vi "OverlayLibraryIconOnVI.vi"(8 "error in (no error)":errorcluster, 9 "Icon in":refnum<class "Icon.lvclass">, 10 "VI Refnum out":refnum<vi>, 11 "LVClassLibrary":refnum<vi>) -> (0 "error out":errorcluster, 1 "Icon out":refnum<class "Icon.lvclass">, 2 "VI Refnum out":refnum<vi>, 3 "LVClassLibrary":refnum<vi>)   [LabVIEW 2019, in "BlueUtilityScripts.lvlib"]
uses:
  <vilib>/LabVIEW Icon API/lv_icon/Classes/Icon/Icon.lvclass
  <vilib>/LabVIEW Icon API/API_User Layer Data.ctl
  <vilib>/Utility/miscctls.llb/LVPoint32TypeDef.ctl
  <vilib>/picture/picture.llb/imagedata.ctl
  BlueUtilityScripts.lvlib
  <vilib>/LabVIEW Icon API/LabVIEW Icon API.lvlib
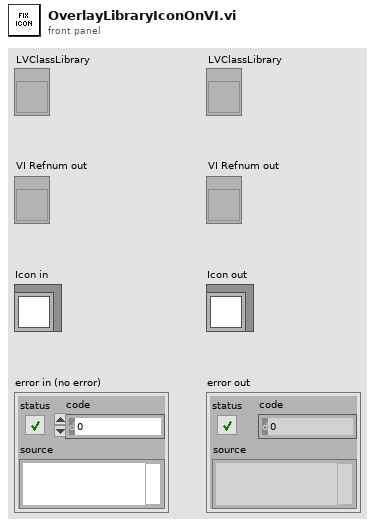
[diagram p1: front panel]
types:
  T1 = typedef "LVPoint32TypeDef.ctl" = cluster{"Horizontal":i32, "Vertical":i32}
  T2 = typedef "LabVIEW Icon API.lvlib/API_User Layer Data.ctl" = cluster{"Layer name":string, "Origin":T1, "Icon image data":T3}
  T3 = typedef "imagedata.ctl" = cluster{"image type":i32, "image depth":i32, "image":u8[], "mask":u8[], "colors":u32[], "Rectangle":cluster{"left":i16, "top":i16, "right":i16, "bottom":i16}}
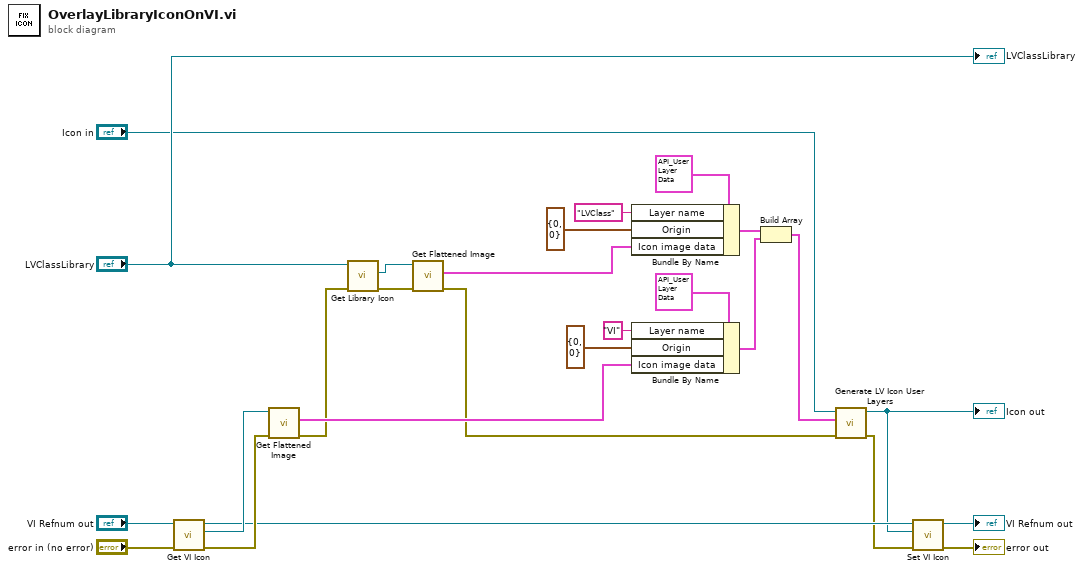
[diagram p0: block diagram]
diagram:
  n1 = call <vilib>:"Get VI Icon.vi"("error in (no error)"="error in (no error)", "VI Refnum in"="VI Refnum out") -> ("error out"=w12:errorcluster, "Icon"=w26:refnum<class "Icon.lvclass">, "VI Refnum out"=w5:refnum<vi>)  [unwired: 7 in]
  n2 = call <vilib>:"Get Flattened Image.vi"("error in (no error)"=w12, "lv_icon.lvlib:Icon.lvclass in"=w26) -> ("error out"=w10:errorcluster, "Color Image"=w15:T3)  [unwired: 6 in, 2 out]
  n3 = call <vilib>:"Get Library Icon.vi"("error in (no error)"=w10, "Library Refnum in"="LVClassLibrary") -> ("error out"=w11:errorcluster, "Icon"=w25:refnum<class "Icon.lvclass">)  [unwired: 7 in, 1 out]
  n4 = call <vilib>:"Get Flattened Image.vi"("error in (no error)"=w11, "lv_icon.lvlib:Icon.lvclass in"=w25) -> ("error out"=w9:errorcluster, "Color Image"=w19:T3)  [unwired: 6 in, 2 out]
  n5 = Bundle By Name(cluster=T2 {"Layer name"="", "Origin"={"Horizontal"=0, "Vertical"=0}, "Icon image data"={"image type"=0, "image depth"=0, "image"=[], "mask"=[], "colors"=[], "Rectangle"={"left"=0, "top"=0, "right"=0, "bottom"=0}}} ("User layer"), "Layer name"="LVClass", "Origin"=T1 {"Horizontal"=0, "Vertical"=0}, "Icon image data"=w19) -> (w21:T2)
  n6 = Bundle By Name(cluster=T2 {"Layer name"="", "Origin"={"Horizontal"=0, "Vertical"=0}, "Icon image data"={"image type"=0, "image depth"=0, "image"=[], "mask"=[], "colors"=[], "Rectangle"={"left"=0, "top"=0, "right"=0, "bottom"=0}}} ("User layer"), "Layer name"="VI", "Origin"=T1 {"Horizontal"=0, "Vertical"=0}, "Icon image data"=w15) -> (w14:T2)
  n7 = Build Array(w21, w14) -> (w20:T2[])
  n8 = call <vilib>:"Generate LV Icon User Layers.vi"("error in (no error)"=w9, "User layers"=w20, "Icon in"="Icon in") -> ("error out"=w4:errorcluster, "Icon out"=w3:refnum<class "Icon.lvclass">)  [unwired: 7 in]
  "Icon out" <- w3
  n9 = call <vilib>:"Set VI Icon.vi"("error in (no error)"=w4, "Icon"=w3, "VI Refnum in"=w5) -> ("error out"=→"error out":errorcluster, "VI Refnum out"=→"VI Refnum out":refnum<vi>)  [unwired: 7 in]
  "LVClassLibrary" <- "LVClassLibrary"
